vi "ZDS1104 Init.vi"(8 "错误输入":errorcluster, 11 "MyIndex":u8) -> (0 "error out":errorcluster caption="错误输出", 3 "ok?":bool)   [LabVIEW 2015]
uses:
  ZhiYuan ZDS Series for TCP/ZhiYuan ZDS Series for TCP.lvlib
panel:
  out "VISA":refnum<visa-resource-name> caption="VISA资源名称输出"
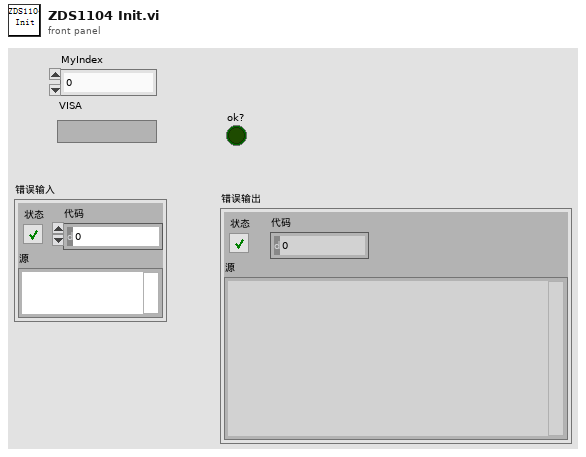
[diagram p1: front panel]
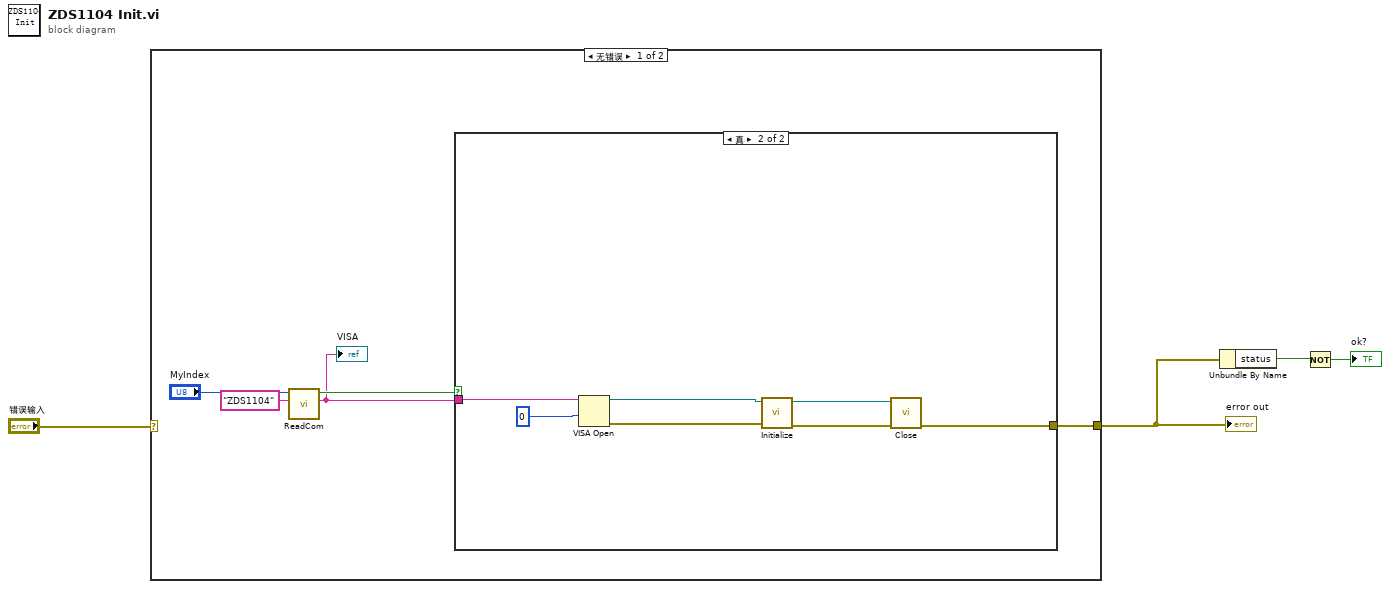
[diagram p0: block diagram]
diagram:
  n1 = case shown="无错误" "错误输入" {
    selector: "错误输入" -> [_ w17]
    tunnel: [w9 w17] -> w2
    frame No Error {
      n2 = call "ReadCom.vi"("仪器名称"="ZDS1104", "MyIndex"="MyIndex") -> ("COM"=w5:string, "OK?"=w6:bool)  [unwired: 7 in, 1 out]
      "VISA" <- w5
      n3 = case shown="真" w6 {
        tunnel: [_ w14] -> w9
        tunnel: w5 -> [_ w15]
        frame False {
        }
        frame True {
          n4 = VISA Open(access mode=u32 0, VISA resource name=w15) -> (VISA resource name=w13:refnum<visa-resource-name>, error out=w12:errorcluster)  [unwired: 3 in]
          n5 = call "Initialize.vi"("error in (no error)"=w12, "VISA resource name"=w13) -> ("error out"=w11:errorcluster, "VISA resource name out"=w10:refnum<visa-resource-name>)  [unwired: 8 in]
          n6 = call "Close.vi"("error in (no error)"=w11, "VISA resource name"=w10) -> ("error out"=w14:errorcluster)  [unwired: 9 in]
        }
      }
    }
    frame Error {
    }
  }
  "error out" <- w2
  n7 = Unbundle By Name(w2) -> ("status"=w4:bool)
  n8 = Not(x=w4) -> (.not. x?=→"ok?":bool)
